vi "SendImageOverTCP.vi"(8 "error in (no error)":errorcluster, 11 "Image":T1) -> (0 "error out":errorcluster)   [LabVIEW 2019]
uses:
  <vilib>/vision/Image Controls.llb/IMAQ Image.ctl
panel:
  out "data out":string
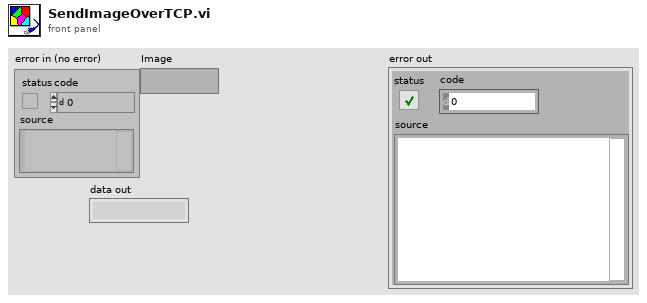
[diagram p1: front panel]
types:
  T1 = typedef "IMAQ Image.ctl" = refnum<image>
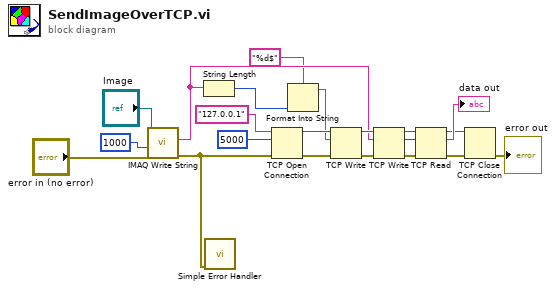
[diagram p0: block diagram]
diagram:
  n1 = call-poly "IMAQ Write String"("error in (no error)"="error in (no error)", "Image Quality"=u32 1000, "Image"="Image") -> ("error out"=w2:errorcluster, "FileString"=w9:string)  [unwired: 6 in, 1 out]
  n2 = String Length(string=w9) -> (length=w8:i32)
  n3 = call <vilib>:"Simple Error Handler.vi"("error in (no error)"=w2) -> ()  [unwired: 4 in, 5 out]
  n4 = TCP Open Connection(address="127.0.0.1", remote port or service name=u16 5000, error in (no error)=w2) -> (connection ID=w19:refnum<k5>, error out=w18:errorcluster)  [unwired: 2 in]
  n5 = Format Into String(format string="%d$", w8) -> (resulting string=w7:string)  [unwired: 2 in, 1 out]
  n6 = TCP Write(connection ID=w19, data in=w7, error in (no error)=w18) -> (connection ID out=w14:refnum<k5>, error out=w13:errorcluster)  [unwired: 1 in, 1 out]
  n7 = TCP Write(connection ID=w14, data in=w9, error in (no error)=w13) -> (connection ID out=w12:refnum<k5>, bytes written=w11:i32, error out=w10:errorcluster)  [unwired: 1 in]
  n8 = TCP Read(connection ID=w12, bytes to read=w11, error in (no error)=w10) -> (connection ID out=w15:refnum<k5>, data out=→"data out":string, error out=w16:errorcluster)  [unwired: 2 in]
  n9 = TCP Close Connection(connection ID=w15, error in (no error)=w16) -> (error out=→"error out":errorcluster)  [unwired: 1 in, 1 out]
